vi "Write_Current_Row_to_log_file.vi"(0 "Current Time":dbl, 1 "Channel Names":string[](array[string]), 2 "Channel Values":string[](array[string]), 3 "Comments":string[](array[string]), 4 "User added comment":string) -> (7 "File Updated?":bool)   [LabVIEW 2015]
uses:
  Anemometry/Anemometry Sub Vis/Globals/Preference_global.vi
  Anemometry/Anemometry Sub Vis/Globals/Constants_global.vi
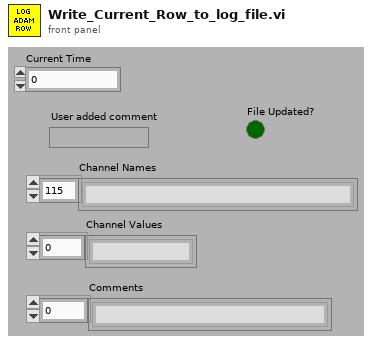
[diagram p1: front panel]
types:
  T1 = typedef "LVDateTimeRec.ctl" = cluster{"fractional second":dbl, "second":i32, "minute":i32, "hour":i32, "day of month":i32, "month":i32, "year":i32, "day of week":i32, "day of year":i32, "DST":i32}
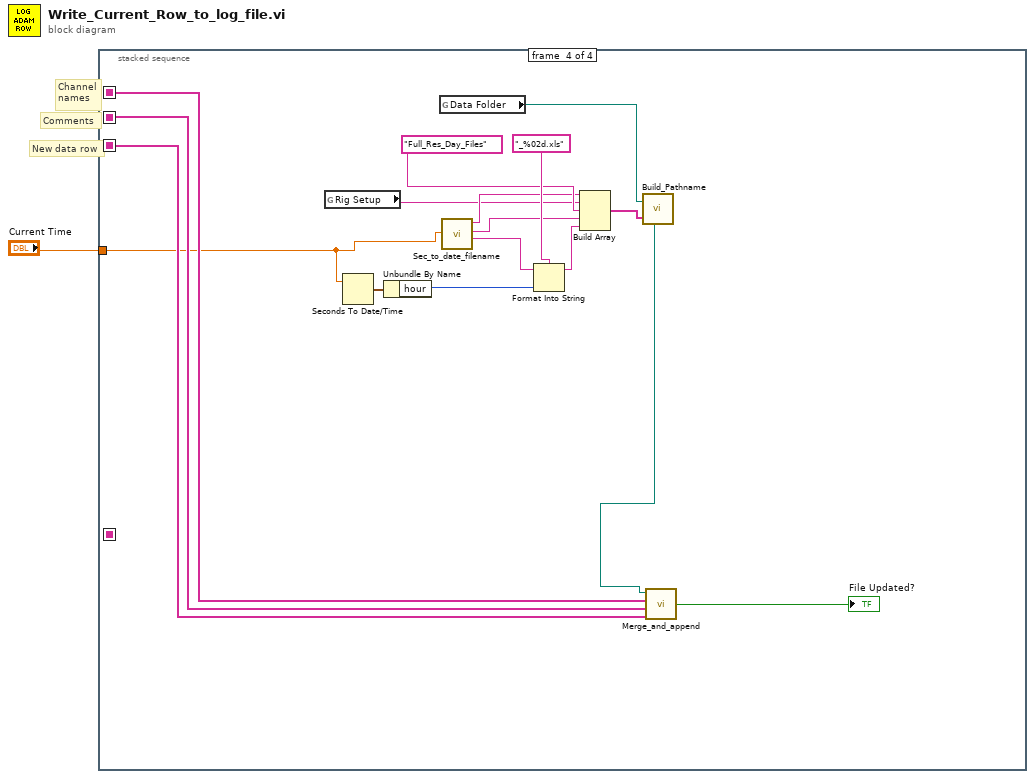
[diagram p0: block diagram]
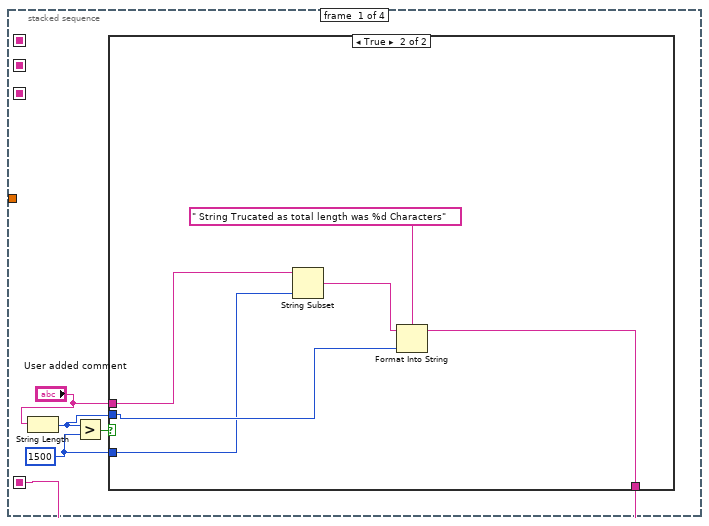
[diagram p2: hidden frame]
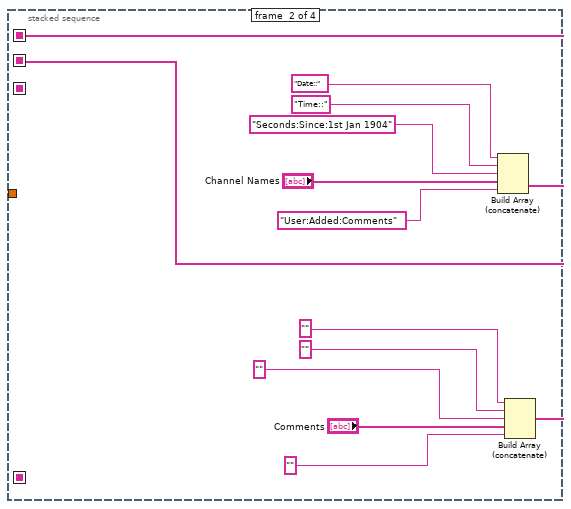
[diagram p4: hidden frame]
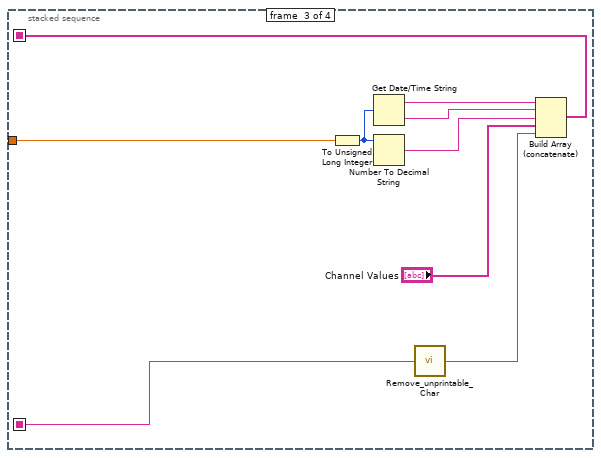
[diagram p5: hidden frame]
diagram:
  # "Comments"
  # "New data row"
  # "Channel\nnames"
  n1 = stacked-sequence {
    seq-local: [_ w22 _ _] -> [_ _ _ w51]
    seq-local: [_ _ w30 _] -> [_ _ _ w49]
    seq-local: [_ w16 _ _] -> [_ _ _ w50]
    seq-local: [w5 _ _ _] -> [_ _ w28 _]
    tunnel: "Current Time" -> [_ _ w26 w36]
    frame #0 {
      w3 = 1500 ("y")
      n2 = String Length(string="User added comment") -> (length=w2:i32)
      n3 = Greater?(x=w2, y=w3) -> (0:w6:bool)
      n4 = case shown="True" w6 {
        tunnel: [w7 w8] -> w5
        tunnel: "User added comment" -> [w7 w13]
        tunnel: w3 -> [_ w9]
        tunnel: w2 -> [_ w12]
        frame False {
        }
        frame True {
          n5 = String Subset(string=w13, length (rest)=w9) -> (substring=w11:string)  [unwired: 1 out]
          n6 = Format Into String(format string=" String Trucated as total length was %d Characters", initial string=w11, w12) -> (resulting string=w8:string)  [unwired: 1 in, 1 out]
        }
      }
    }
    frame #1 {
      n7 = Build Array (concatenate)("Date::", "Time::", "Seconds:Since:1st Jan 1904", "Channel Names", "User:Added:Comments") -> (w22:string[])
      n8 = Build Array (concatenate)("", "", "", "Comments", "") -> (w16:string[])
    }
    frame #2 {
      n9 = To Unsigned Long Integer(number=w26) -> (unsigned 32bit integer=w31:u32)
      n10 = Get Date/Time String(seconds (now)=w31) -> (date string=w34:string, time string=w33:string)  [unwired: 2 out]
      n11 = Number To Decimal String(number=w31) -> (decimal integer string=w32:string)  [unwired: 1 out]
      n12 = call "Remove_unprintable_Char.vi"("Input String"=w28) -> ("Output String"=w29:string)
      n13 = Build Array (concatenate)(w34, w33, w32, "Channel Values", w29) -> (w30:string[])
    }
    frame #3 {
      n14 = global read "Preference_global.vi" "Rig Setup"() -> (w40:string)
      n15 = Seconds To Date/Time(time stamp (now)=w36) -> (date time rec=w41:T1)  [unwired: 1 in]
      n16 = Unbundle By Name(w41) -> ("hour"=w35:i32)
      n17 = global read "Constants_global.vi" "Data Folder"() -> (w39:path)
      n18 = call "Sec_to_date_filename.vi"("seconds"=w36) -> ("Year"=w43:string, "Month"=w42:string, "Day"=w47:string)  [unwired: 1 out]
      n19 = Format Into String(format string="_%02d.xls", initial string=w47, w35) -> (resulting string=w46:string)  [unwired: 1 in, 1 out]
      n20 = Build Array(w43, w40, "Full_Res_Day_Files" ("Input Element"), w42, w46) -> (w38:string[])
      n21 = call "Build_Pathname.vi"("PathElements"=w38, "PathnameIn"=w39) -> ("AppendedPath"=w37:path)
      n22 = call "Merge_and_append.vi"("New Row"=w49, "Comments"=w50, "Channel Names"=w51, "Path name"=w37) -> ("File Updated?"=→"File Updated?":bool)
    }
  }
